vi "Draw Indentify line.vi"(6 "Refs":T1, 8 "error in (no error)":errorcluster, 9 "Coords-end":T3, 11 "PlotAreaBounds":T2) -> (0 "error out":errorcluster, 3 "picture":picture)   [LabVIEW 2021, in "RocketPlot.lvlib"]
uses:
  RocketPlot.lvlib
  <vilib>/Utility/miscctls.llb/LVPoint32TypeDef.ctl
  <vilib>/Utility/miscctls.llb/LVRectTypeDef.ctl
  TypeDefs/Plot UI references.ctl
  Classes/RocketPlotHandle/RocketPlotHandle.lvclass
  <userlib>/bjustice/TipStripOOPanel/Classes/TipPanelHandle/TipPanelHandle.lvclass
  TypeDefs/Plot top row.ctl
  Search for oldest time to keep DBL.vi
  <vilib>/gmath/interp.llb/Interpolate 1D.vi
  <vilib>/picture/picture.llb/Get Text Rect.vi
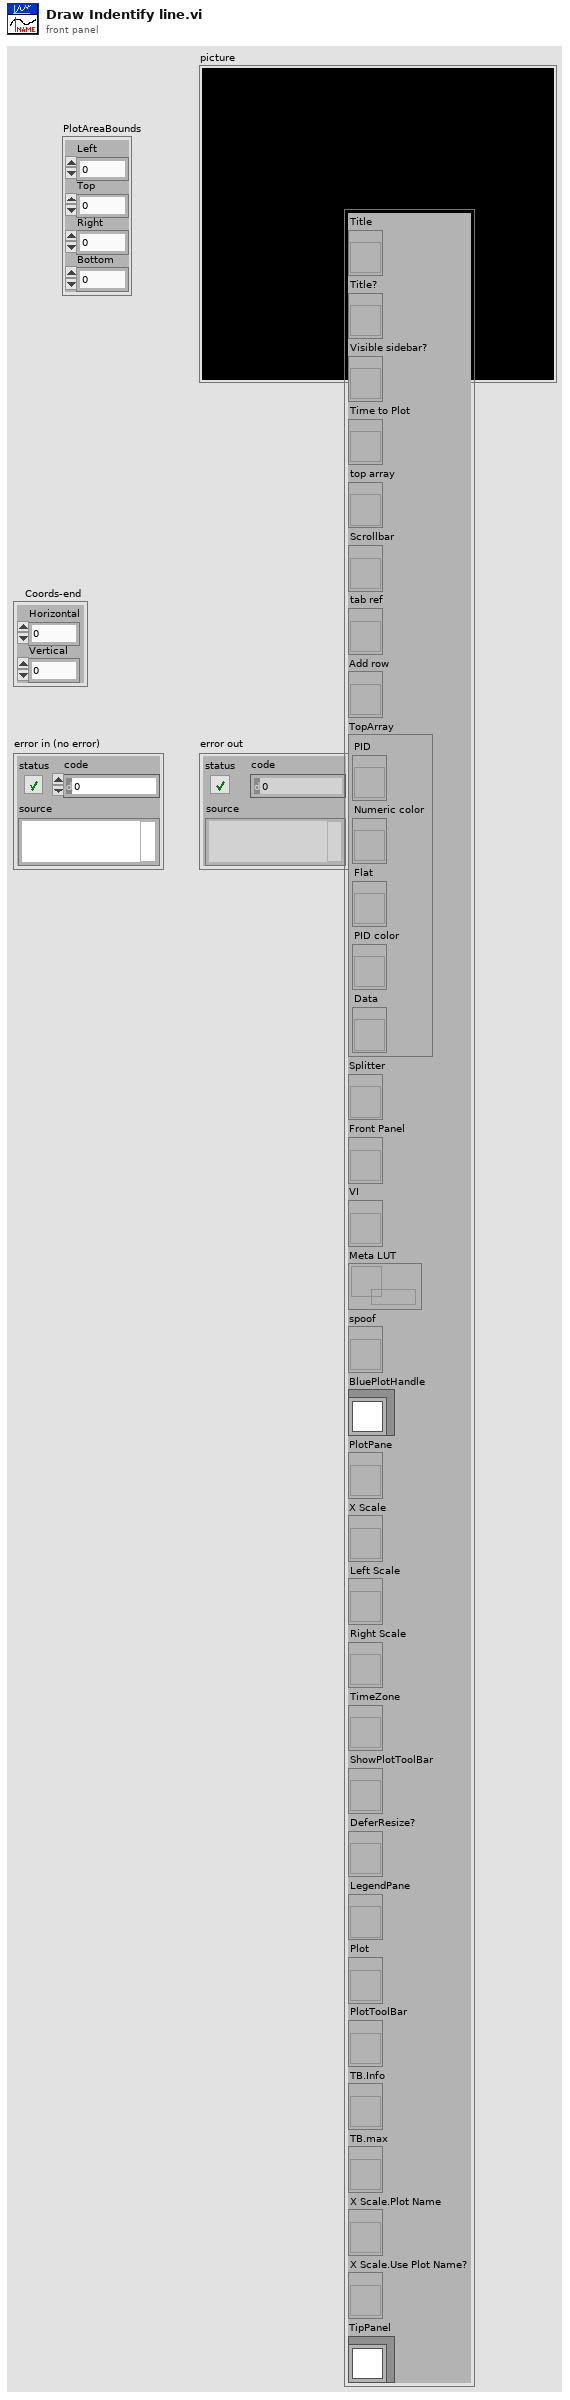
[diagram p1: front panel]
types:
  T1 = typedef "RocketPlot.lvlib/Plot UI references.ctl" = cluster{"Title":refnum<vi>, "Title?":refnum<vi>, "Visible sidebar?":refnum<vi>, "Time to Plot":refnum<vi>, "top array":refnum<vi>, "Scrollbar":refnum<vi>, "tab ref":refnum<vi>, "Add row":refnum<vi>, "TopArray":cluster{"PID":refnum<vi>, "Numeric color":refnum<vi>, "Flat":refnum<vi>, "PID color":refnum<vi>, "Data":refnum<vi>}, "Splitter":refnum<vi>, "Front Panel":refnum<vi>, "VI":refnum<vi>, "Meta LUT":refnum<data-value>, "spoof":refnum<vi>, "BluePlotHandle":refnum<class "RocketPlotHandle.lvclass">, "PlotPane":refnum<vi>, "X Scale":refnum<vi>, "Left Scale":refnum<vi>, "Right Scale":refnum<vi>, "TimeZone":refnum<vi>, "ShowPlotToolBar":refnum<vi>, "DeferResize?":refnum<vi>, "LegendPane":refnum<vi>, "Plot":refnum<vi>, "PlotToolBar":refnum<vi>, "TB.Info":refnum<vi>, "TB.max":refnum<vi>, "X Scale.Plot Name":refnum<vi>, "X Scale.Use Plot Name?":refnum<vi>, "TipPanel":refnum<class "TipPanelHandle.lvclass">}
  T2 = typedef "LVRectTypeDef.ctl" = cluster{"Left":i16, "Top":i16, "Right":i16, "Bottom":i16}
  T3 = typedef "LVPoint32TypeDef.ctl" = cluster{"Horizontal":i32, "Vertical":i32}
  T4 = cluster{"left":i16, "top":i16, "right":i16, "bottom":i16}
  T5 = cluster{"Width":u16, "Style":enum32{"Solid", "Dash", "Dot", "DashDot", "DashDotDot"}}
  T6 = typedef "StokePlot.lvlib/Plot top row.ctl" = cluster{"PID":string, "index":i32, "PID color":u32, "right axis?":bool, "Flatline?":bool, "Numeric color":u32, "Data":string, "Flat":string}
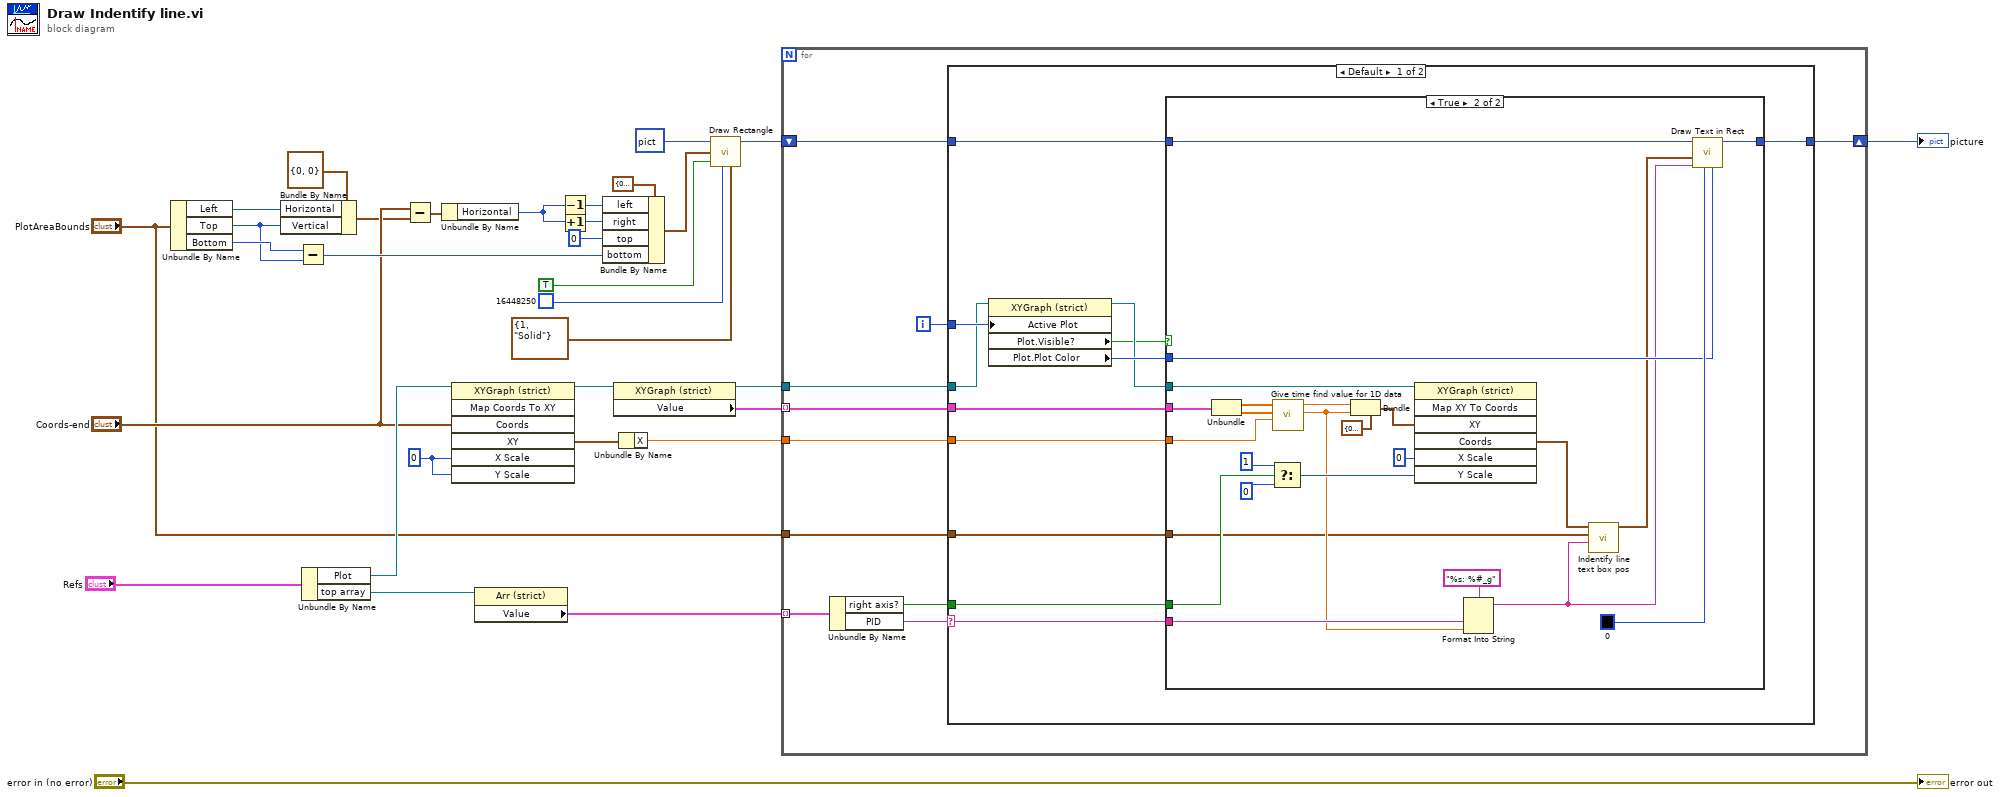
[diagram p0: block diagram]
diagram:
  w6 = 0 ("X Scale")
  n1 = Unbundle By Name("PlotAreaBounds") -> ("Left"=w30:i16, "Top"=w20:i16, "Bottom"=w21:i16)
  n2 = Bundle By Name(cluster=T3 {"Horizontal"=0, "Vertical"=0} ("Coords"), "Horizontal"=w30, "Vertical"=w20) -> (w2:T3)
  n3 = Subtract(x=w21, y=w20) -> (x-y=w19:i16)
  n4 = Unbundle By Name("Refs") -> ("Plot"=w8:refnum<vi>, "top array"=w15:refnum<vi>)
  n5 = Subtract(x="Coords-end", y=w2) -> (x-y=w3:T3)
  n6 = Unbundle By Name(w3) -> ("Horizontal"=w25:i32)
  n7 = invoke class="XYGraph (strict)" method="Map Coords To XY"(reference=w8, "Coords"="Coords-end", "X Scale"=w6, "Y Scale"=w6) -> (reference out=w9:refnum<vi>, "XY"=w5:cluster{"X":dbl, "Y":dbl})  [unwired: 3 in, 5 out]
  n8 = property class="Arr (strict)"(reference=w15) -> ("Value"=w14:T6[])  [unwired: 1 in, 2 out]
  n9 = Decrement(x=w25) -> (x-1=w26:i32)
  n10 = Increment(x=w25) -> (x+1=w27:i32)
  n11 = Bundle By Name(cluster=T4 {"left"=0, "top"=0, "right"=0, "bottom"=0} ("rect"), "left"=w26, "right"=w27, "top"=i16 0 ("x-y"), "bottom"=w19) -> (w23:T4)
  n12 = property class="XYGraph (strict)"(reference=w9) -> (reference out=w10:refnum<vi>, "Value"=w11:cluster{dbl[], "Data":dbl[]}[])  [unwired: 1 in, 1 out]
  n13 = Unbundle By Name(w5) -> ("X"=w4:dbl)
  n14 = call <vilib>:"Draw Rectangle.vi"("picture"=picture data[5B], "rect"=w23, "fill?(F)"=TRUE, "color(black)"=u32 16448250, "pen"=T5 {"Width"=1, "Style"=enum."Solid"}) -> ("new picture"=w13:picture)  [unwired: 4 in]
  n15 = for {
    tunnel: w10 -> [w35]
    tunnel: w14 -> [w42] mode=indexing
    tunnel: "PlotAreaBounds" -> [w34]
    shift-right: [w39] -> w12
    shift-left: w13 -> [w40]
    tunnel: w11 -> [w37] mode=indexing
    tunnel: w4 -> [w36]
    i -> [w38]
    n16 = Unbundle By Name(w42) -> ("right axis?"=w41:bool, "PID"=w33:string)
    n17 = case shown="Default" w33 {
      selector: w33 -> [w47 _]
      tunnel: w41 -> [w54 _]
      tunnel: w40 -> [w53 w80]
      tunnel: [w52 w80] -> w39
      tunnel: w38 -> [w51 _]
      tunnel: w37 -> [w50 _]
      tunnel: w36 -> [w48 _]
      tunnel: w35 -> [w45 _]
      tunnel: w34 -> [w49 _]
      frame Default {
        n18 = property class="XYGraph (strict)"(reference=w45, "Active Plot"=w51) -> (reference out=w44:refnum<vi>, "Plot.Visible?"=w43:bool, "Plot.Plot Color"=w46:u32)  [unwired: 1 in, 1 out]
        n19 = case shown="True" w43 {
          tunnel: w54 -> [_ w79]
          tunnel: w53 -> [w55 w76]
          tunnel: [w55 w75] -> w52
          tunnel: w50 -> [_ w74]
          tunnel: w49 -> [_ w60]
          tunnel: w48 -> [_ w57]
          tunnel: w47 -> [_ w65]
          tunnel: w46 -> [_ w63]
          tunnel: w44 -> [_ w62]
          frame False {
          }
          frame True {
            n20 = Unbundle(w74) -> (w73:dbl[], "Data"=w72:dbl[])
            n21 = Select(t=1 ("Y Scale"), s=w79, f=0 ("Y Scale")) -> (s? t:f=w68:i32)
            n22 = call "Give time find value for 1D data.vi"("Time (lookup)"=w57, "Data"=w72, "Time (s)"=w73) -> ("data"=w64:dbl, "time"=w56:dbl)  [unwired: 7 in]
            n23 = Bundle(cluster=cluster{"X":dbl, "Y":dbl} {"X"=0.0, "Y"=0.0} ("XY"), "X"=w56, "Y"=w64) -> (w70:cluster{"X":dbl, "Y":dbl})
            n24 = invoke class="XYGraph (strict)" method="Map XY To Coords"(reference=w62, "XY"=w70, "X Scale"=0, "Y Scale"=w68) -> ("Coords"=w61:T3)  [unwired: 3 in, 6 out]
            n25 = Format Into String(format string="%s: %#_g", w65, w64) -> (resulting string=w59:string)  [unwired: 2 in, 1 out]
            n26 = call "Indentify line text box pos.vi"("text"=w59, "PlotAreaBounds"=w60, "Coords"=w61) -> ("rect"=w58:T4)  [unwired: 7 in, 1 out]
            n27 = call <vilib>:"Draw Text in Rect.vi"("BG color(transparent)"=w63, "text color(black)"=u32 0 ("BG color(transparent)"), "text"=w59, "rect"=w58, "picture"=w76) -> ("new picture"=w75:picture)  [unwired: 6 in]
          }
        }
      }
      frame "" {
      }
    }
  }
  "picture" <- w12
  "error out" <- "error in (no error)"
